vi "DP-Options Dialog.vi"(7 "Parent VI":refnum<vi>, 9 "Advanced options":T1, 10 "StimGen":T2, 11 "Advanced?":bool) -> (1 "Advanced options out":T1, 2 "StimGen out":T2, 3 "Cancelled?":bool=TRUE)   [LabVIEW 2020]
doc: "Use this template to create a dialog box with event handling."
uses:
  Typedefs/DP-StimGen.ctl
  Typedefs/DP-Advanced Options.ctl
panel:
  in  "Spec avgs":string
  in  "Time avgs":string
  in  "Override recal check":bool caption="Ignore recalibration error"
  in  "Buffer length (ms)":dbl
  in  "Sampling rate (Hz)":dbl
  in  "Cancel":bool
  in  "OK":bool
  # "I/O Parameters"
  # "Advanced"
  # "Recalibration"
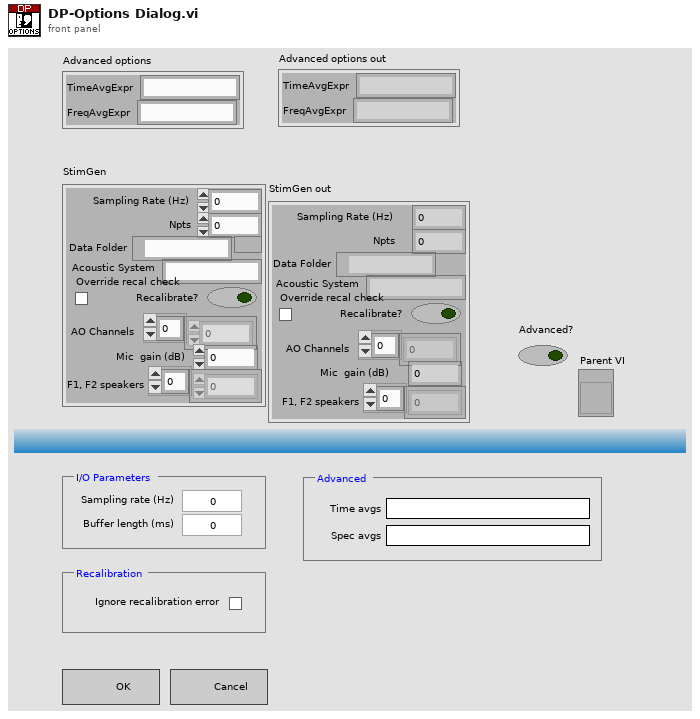
[diagram p1: front panel]
types:
  T1 = typedef "DP-Advanced Options.ctl" = cluster{"TimeAvgExpr":string, "FreqAvgExpr":string}
  T2 = typedef "DP-StimGen.ctl" = cluster{"Sampling Rate (Hz)":dbl, "Npts":i32, "Data Folder":path, "Acoustic System":string, "Recalibrate?":bool, "AO Channels":i32[], "Mic  gain (dB)":dbl, "F1, F2 speakers":i32[], "Override recal check":bool}
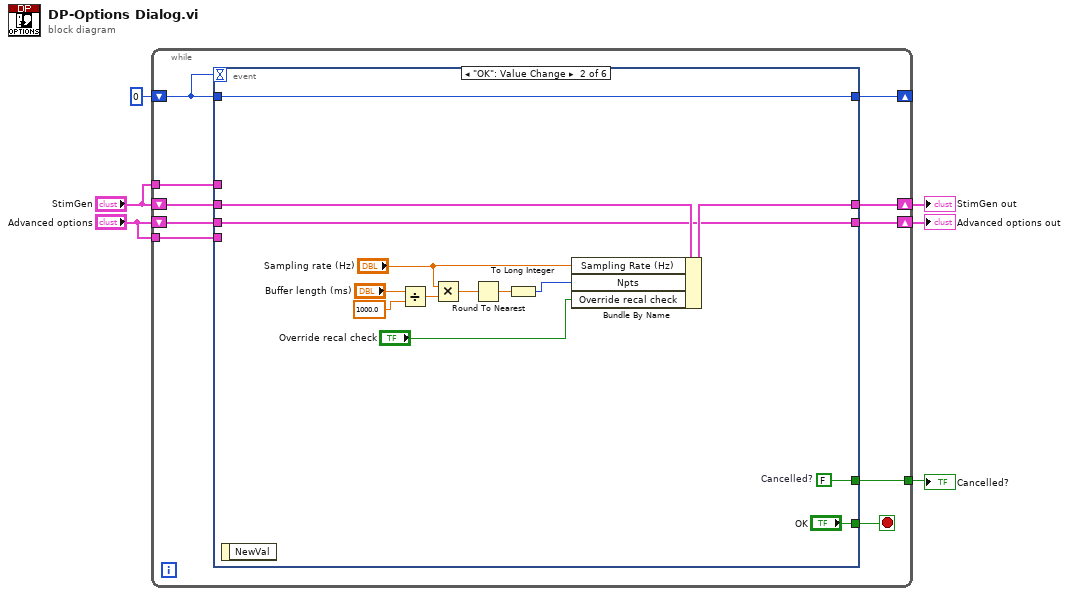
[diagram p0: block diagram]
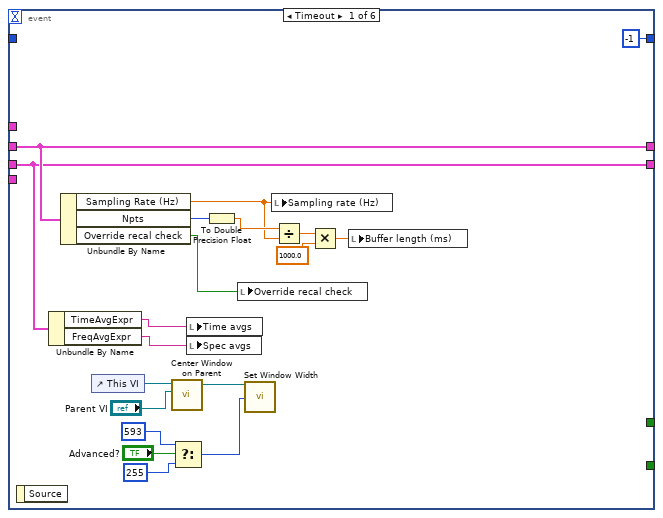
[diagram p2: hidden frame]
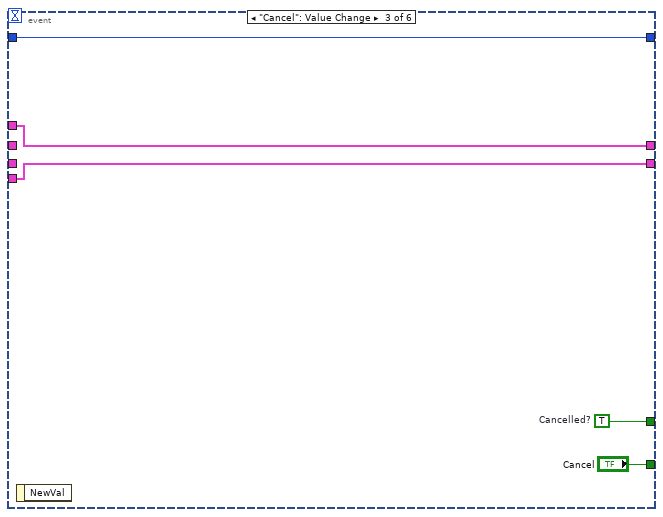
[diagram p3: hidden frame]
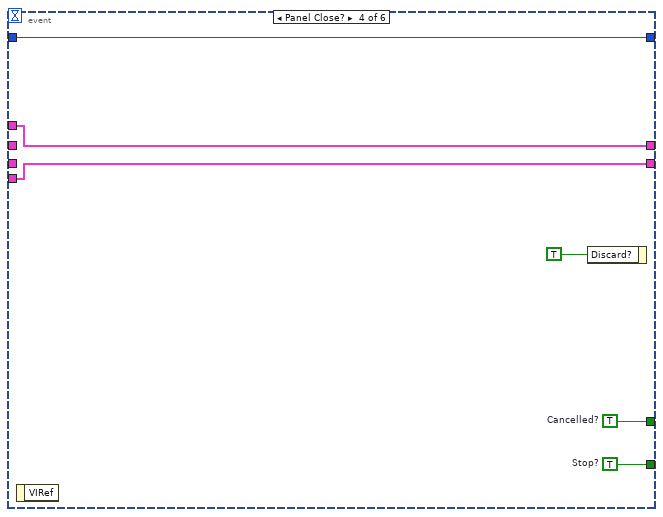
[diagram p4: hidden frame]
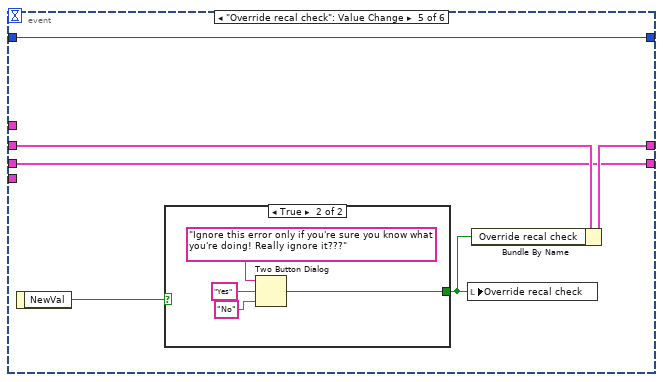
[diagram p5: hidden frame]
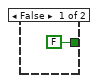
[diagram p6: hidden frame]
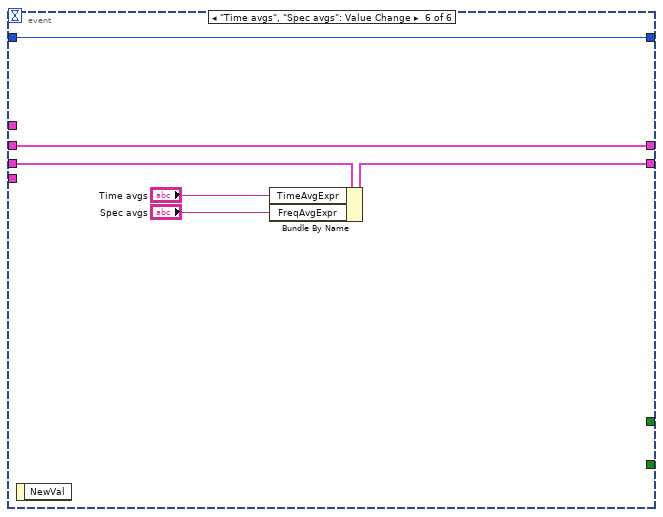
[diagram p7: hidden frame]
diagram:
  n1 = while {
    tunnel: [w15] -> w6
    shift-right: [w14] -> _
    shift-left: 0 -> [w10]
    tunnel: "StimGen" -> [w11]
    shift-right: [w12] -> w4
    shift-left: "StimGen" -> [w13]
    shift-right: [w8] -> w1
    shift-left: "Advanced options" -> [w9]
    tunnel: "Advanced options" -> [w7]
    stop <- w16 stop-if-true
    n2 = event shown="[1] \"OK\": Value Change" {
      selector: _ -> [_ _ _ _ _ _]
      dyn-events: _ -> [_ _ _ _ _ _]
      timeout: w10 -> [_ _ _ _ _ _]
      tunnel: [_ "OK" "Cancel" w59 _ _] -> w16
      tunnel: [_ w49 w54 w58 _ _] -> w15
      tunnel: [-1 w37 w51 w57 w62 w77] -> w14
      tunnel: w13 -> [w27 w42 _ _ w66 w75]
      tunnel: [w27 w39 w52 w56 w64 w75] -> w12
      tunnel: w11 -> [_ _ w52 w56 _ _]
      tunnel: w10 -> [_ w37 w51 w57 w62 w77]
      tunnel: w9 -> [w19 w36 _ _ w61 w76]
      tunnel: [w19 w36 w50 w55 w61 w74] -> w8
      tunnel: w7 -> [_ _ w50 w55 _ _]
      event Timeout {
        n3 = event-data() -> ()  [unwired: 1 in, 1 out]
        n4 = Unbundle By Name(w19) -> ("TimeAvgExpr"=w18:string, "FreqAvgExpr"=w17:string)
        n5 = Unbundle By Name(w27) -> ("Sampling Rate (Hz)"=w32:dbl, "Npts"=w34:i32, "Override recal check"=w28:bool)
        n6 = control-ref of="This VI"() -> (w26:refnum<vi>)
        n7 = call "Center Window on Parent.vi"("Parent VI"="Parent VI", "VI in"=w26) -> ("VI out"=w24:refnum<vi>)  [unwired: 8 in, 1 out]
        n8 = Select(t=593, s="Advanced?", f=255) -> (s? t:f=w21:i32)
        n9 = local write "Time avgs"(w18) -> ()
        n10 = local write "Spec avgs"(w17) -> ()
        n11 = To Double Precision Float(number=w34) -> (double precision float=w33:dbl)
        n12 = local write "Override recal check"(w28) -> ()
        n13 = call "Set Window Width.vi"("VI in"=w24, "Width"=w21) -> ()  [unwired: 12 in, 2 out]
        n14 = local write "Sampling rate (Hz)"(w32) -> ()
        n15 = Divide(x=w33, y=w32) -> (x/y=w31:dbl)
        n16 = Multiply(x=w31, y=1000.0) -> (x*y=w29:dbl)
        n17 = local write "Buffer length (ms)"(w29) -> ()
      }
      event "OK": Value Change {
        w49 = FALSE  # Cancelled?
        n18 = event-data() -> ()  [unwired: 1 in, 1 out]
        n19 = Divide(x="Buffer length (ms)", y=1000.0) -> (x/y=w45:dbl)
        n20 = Multiply(x="Sampling rate (Hz)", y=w45) -> (x*y=w44:dbl)
        n21 = Round To Nearest(number=w44) -> (nearest integer value=w43:dbl)
        n22 = To Long Integer(number=w43) -> (32bit integer=w40:i32)
        n23 = Bundle By Name(cluster=w42, "Sampling Rate (Hz)"="Sampling rate (Hz)", "Npts"=w40, "Override recal check"="Override recal check") -> (w39:T2)
      }
      event "Cancel": Value Change {
        w54 = TRUE  # Cancelled?
        n24 = event-data() -> ()  [unwired: 1 in, 1 out]
      }
      event Panel Close? {
        w58 = TRUE  # Cancelled?
        w59 = TRUE  # Stop?
        n25 = event-data() -> ()  [unwired: 1 in, 1 out]
        n26 = event-data("Discard?"=TRUE) -> ()  [unwired: 1 in, 1 out]
      }
      event "Override recal check": Value Change {
        n27 = event-data() -> ("NewVal"=w65:bool)  [unwired: 1 in]
        n28 = case shown="True" w65 {
          tunnel: [FALSE ("T button?") w68] -> w63
          frame False {
          }
          frame True {
            n29 = Two Button Dialog(message="Ignore this error only if you're sure you know what you're doing! Really ignore it???", 1:"No" ("F button name (\"Cancel\")"), 2:"Yes" ("T button name (\"OK\")")) -> (T button?=w68:bool)
          }
        }
        n30 = local write "Override recal check"(w63) -> ()
        n31 = Bundle By Name(cluster=w66, "Override recal check"=w63) -> (w64:T2)
      }
      event "Time avgs", "Spec avgs": Value Change {
        n32 = event-data() -> ()  [unwired: 1 in, 1 out]
        n33 = Bundle By Name(cluster=w76, "TimeAvgExpr"="Time avgs", "FreqAvgExpr"="Spec avgs") -> (w74:T1)
      }
    }
  }
  "Cancelled?" <- w6
  "StimGen out" <- w4
  "Advanced options out" <- w1
